vi "init.vi"(8 "error in (no error)":errorcluster, 11 "Soda Actor in":refnum<class "Soda Actor.lvclass">) -> (0 "error out":errorcluster, 3 "Soda Actor out":refnum<class "Soda Actor.lvclass">)   [LabVIEW 2020, in "Soda Actor.lvlib" / "Soda Actor.lvclass"]
uses:
  Soda Actor.lvclass
  Soda Actor.lvclass/Soda Actor.ctl
  <vilib>/Utility/config.llb/Read Key (Double).vi
  <vilib>/Utility/config.llb/Read Key (String).vi
  <vilib>/Utility/config.llb/NI_LVConfig.lvlib
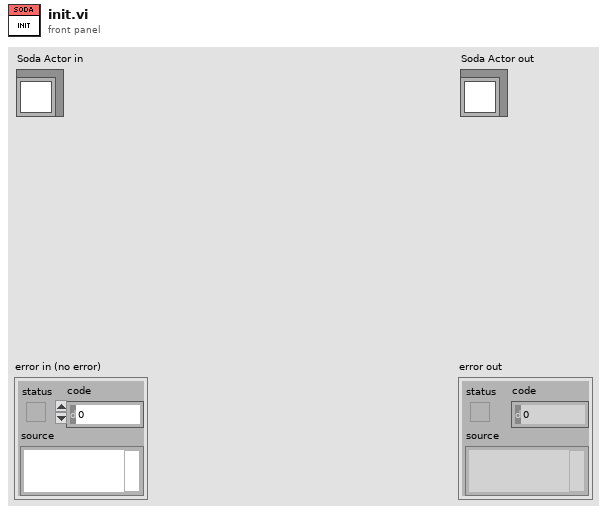
[diagram p1: front panel]
types:
  T1 = typedef "NI_LVConfig.lvlib/Config Data RefNum.ctl" = refnum<k1>
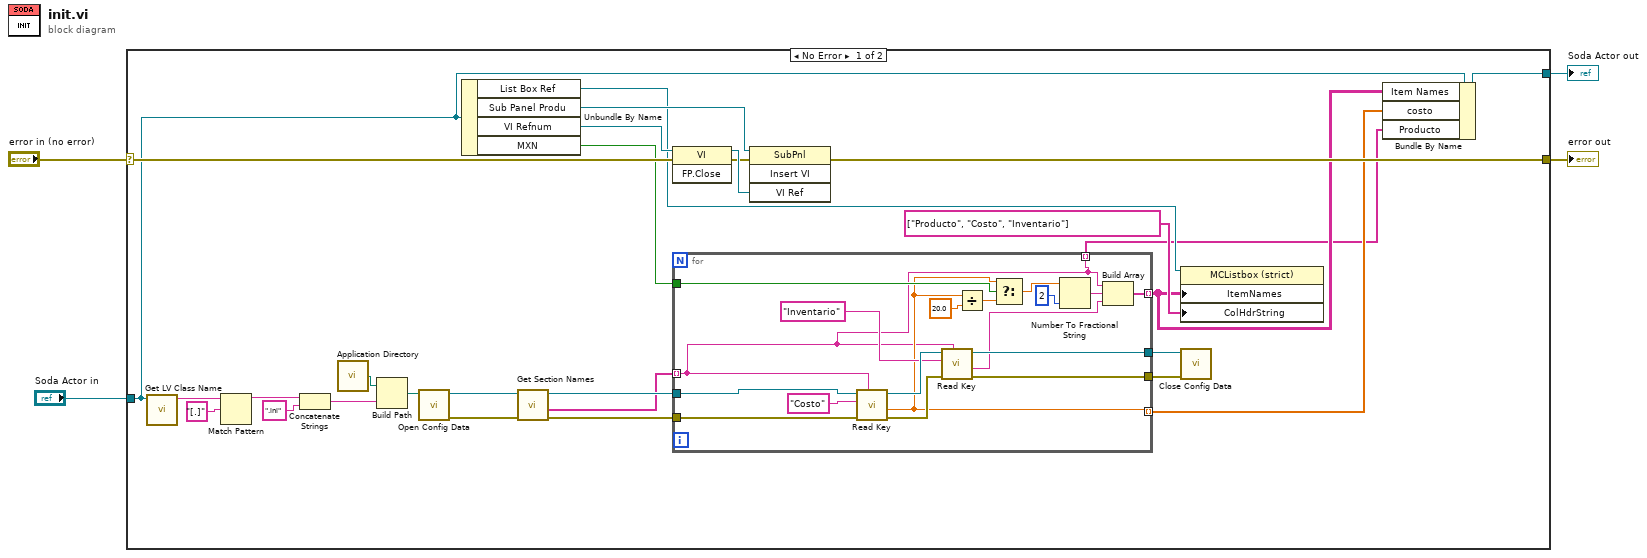
[diagram p0: block diagram]
diagram:
  n1 = case shown="No Error" "error in (no error)" {
    selector: "error in (no error)" -> [w28 w52]
    tunnel: [w27 w52] -> w3
    tunnel: [w8 w51] -> w1
    tunnel: "Soda Actor in" -> [w25 w51]
    frame No Error {
      n2 = call <vilib>:"Get LV Class Name.vi"("object"=w25) -> ("class name"=w18:string)  [unwired: 9 in, 1 out]
      n3 = Match Pattern(string=w18, regular expression="[.]") -> (before substring=w16:string)  [unwired: 1 in, 3 out]
      n4 = Concatenate Strings(w16, ".ini") -> (w23:string)
      n5 = call <vilib>:"Application Directory.vi"() -> ("Application Directory"=w24:path)
      n6 = Build Path(base path=w24, name or relative path=w23) -> (appended path=w21:path)
      n7 = call <vilib>:"Open Config Data.vi"("configuration file path"=w21) -> ("error out"=w14:errorcluster, "refnum"=w15:T1)  [unwired: 8 in, 1 out]
      n8 = Unbundle By Name(w25) -> ("List Box Ref"=w26:refnum<vi>, "Sub Panel Produ"=w32:refnum<vi>, "VI Refnum"=w31:refnum<vi>, "MXN"=w9:bool)
      n9 = call <vilib>:"Get Section Names.vi"("error in (no error)"=w14, "refnum"=w15) -> ("error out"=w12:errorcluster, "section names"=w11:string[], "refnum out"=w13:T1)  [unwired: 7 in]
      n10 = invoke class="VI" method="FP.Close"(reference=w31, error in=w28) -> (reference out=w30:refnum<vi>, error out=w29:errorcluster)  [unwired: 1 in, 1 out]
      n11 = for {
        tunnel: w13 -> [w50]
        tunnel: w12 -> [w49]
        tunnel: [w41] -> w7 mode=indexing
        tunnel: [w45] -> w20
        tunnel: [w46] -> w19
        tunnel: w11 -> [w33] mode=indexing
        tunnel: w9 -> [w38]
        tunnel: [w34] -> w6 mode=indexing
        tunnel: [w33] -> w5 mode=indexing
        n12 = call-poly <vilib>:"Read Key.vi"("section"=w33, "error in (no error)"=w49, "key"="Costo", "refnum"=w50) -> ("error out"=w48:errorcluster, "value"=w34:dbl, "refnum out"=w47:T1)  [unwired: 4 in, 1 out]
        n13 = call-poly <vilib>:"Read Key.vi"("section"=w33, "error in (no error)"=w48, "key"="Inventario", "refnum"=w47) -> ("error out"=w46:errorcluster, "value"=w42:string, "refnum out"=w45:T1)  [unwired: 4 in, 1 out]
        n14 = Divide(x=w34, y=20.0) -> (x/y=w36:dbl)
        n15 = Select(t=w34, s=w38, f=w36) -> (s? t:f=w37:dbl)
        n16 = Number To Fractional String(number=w37, precision (6)=i16 2) -> (F-format string=w40:string)  [unwired: 2 in]
        n17 = Build Array(w33, w40, w42) -> (w41:string[])
      }
      n18 = invoke class="SubPnl" method="Insert VI"(reference=w32, error in=w29, "VI Ref"=w30) -> (error out=w27:errorcluster)  [unwired: 1 in, 3 out]
      n19 = property class="MCListbox (strict)"(reference=w26, "ItemNames"=w7, "ColHdrString"=string[] ["Producto", "Costo", "Inventario"] ("Column Header Strings[]")) -> ()  [unwired: 1 in, 2 out]
      n20 = call <vilib>:"Close Config Data.vi"("error in (no error)"=w19, "refnum"=w20) -> ()  [unwired: 8 in, 2 out]
      n21 = Bundle By Name(cluster=w25, "Item Names"=w7, "costo"=w6, "Producto"=w5) -> (w8:refnum<class "Soda Actor.lvclass">)
    }
    frame Error {
    }
  }
  "error out" <- w3
  "Soda Actor out" <- w1
